vi "WorkorderHandler_CreateScript.vi"(8 "error in (no error)":errorcluster, 11 "reference":T1) -> (0 "error out":errorcluster, 3 "duplicate reference":T1)   [LabVIEW 2011]
uses:
  DataStructures/WorkorderHandler_ObjectReference.ctl
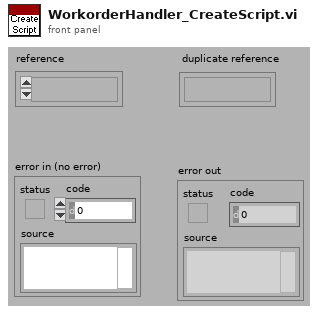
[diagram p1: front panel]
types:
  T1 = typedef "WorkorderHandler_ObjectReference.ctl" = refnum<k1>
  T2 = typedef "WorkorderHandler_ObjectData.ctl" = cluster{"Table":string[][], "Script":string, "Order":string, "No":string, "Time":dbl}
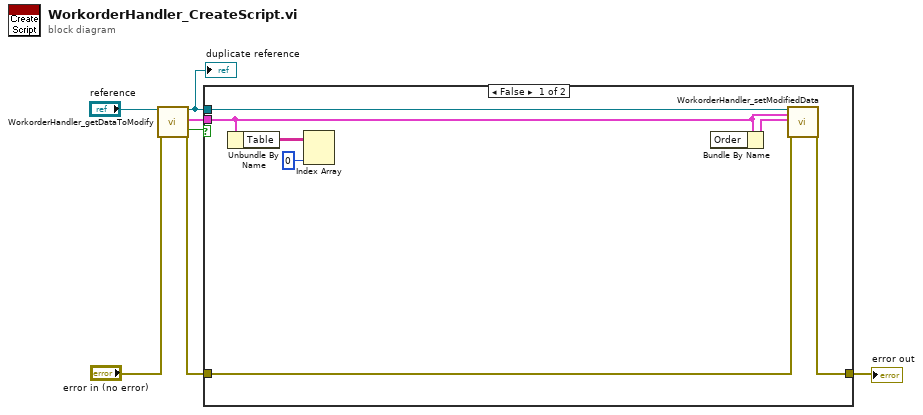
[diagram p0: block diagram]
diagram:
  n1 = call "WorkorderHandler_getDataToModify.vi"("reference"="reference", "error in (no error)"="error in (no error)") -> ("duplicate reference"=w3:T1, "data"=w6:T2, "timed out?"=w1:bool, "error out"=w2:errorcluster)  [unwired: 1 in, 13 out]
  "duplicate reference" <- w3
  n2 = case shown="False" w1 {
    tunnel: [w13 w15] -> w7
    tunnel: w6 -> [w11 _]
    tunnel: w3 -> [w14 _]
    tunnel: w2 -> [w10 w15]
    frame False {
      n3 = Unbundle By Name(w11) -> ("Table"=w9:string[][])
      n4 = Index Array(array=w9, index (col)=0 ("disabled index (col)")) -> ()  [unwired: 1 in, 1 out]
      n5 = Bundle By Name(cluster=w11) -> (w12:T2)  [unwired: 1 in]
      n6 = call "WorkorderHandler_setModifiedData.vi"("reference"=w14, "data (unmodified)"=w11, "data"=w12, "error in (no error)"=w10) -> ("error out"=w13:errorcluster)  [unwired: 15 out]
    }
    frame True {
      # "Error or Timed Out"
    }
  }
  "error out" <- w7
